vi "imuSensor_Init.vi"(8 "error in (no error)":errorcluster, 11 "imuSensor in":refnum<class "imuSensor.lvclass">) -> (0 "error out":errorcluster, 3 "imuSensor out":refnum<class "imuSensor.lvclass">)   [LabVIEW 2020, in "RPI.SenseHat.Sensors.lvlib" / "imuSensor.lvclass"]
uses:
  imuSensor.lvclass
  imuSensor.lvclass/imuSensor.ctl
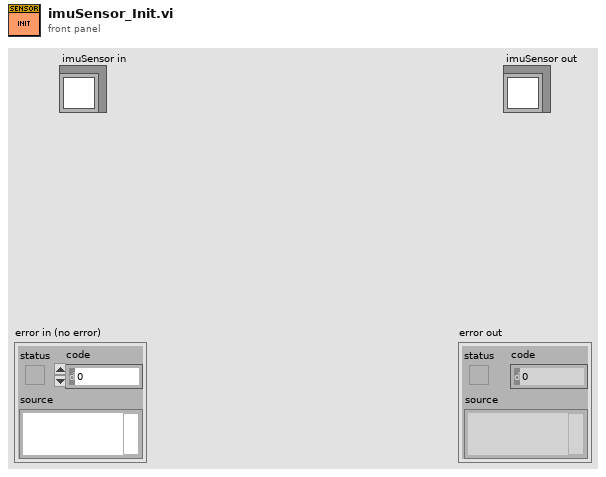
[diagram p1: front panel]
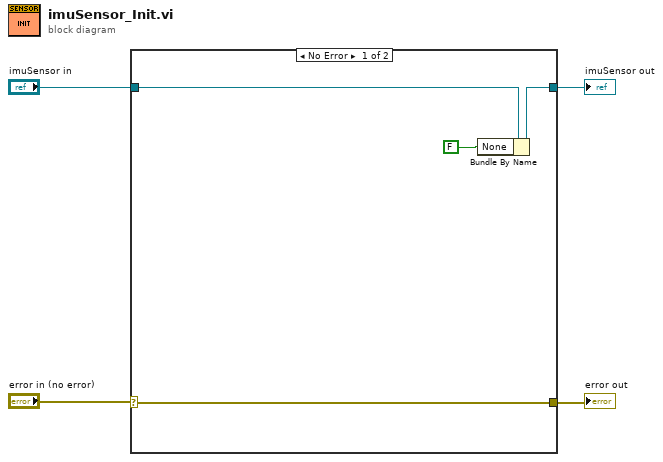
[diagram p0: block diagram]
diagram:
  n1 = case shown="No Error" "error in (no error)" {
    selector: "error in (no error)" -> [w5 w9]
    tunnel: "imuSensor in" -> [w8 w10]
    tunnel: [w7 w10] -> w3
    tunnel: [w5 w9] -> w1
    frame No Error {
      n2 = Bundle By Name(cluster=w8, "None"=FALSE) -> (w7:refnum<class "imuSensor.lvclass">)
    }
    frame Error {
    }
  }
  "imuSensor out" <- w3
  "error out" <- w1
